vi "To Variant.vi"(0 "Obj in":refnum<class "Channel.lvclass">, 11 "error in (no error)":errorcluster) -> (4 "Obj out":refnum<class "Channel.lvclass">, 8 "Array":variant[](array[variant]), 15 "error out":errorcluster)   [LabVIEW 2020, in "Channel.lvclass"]
uses:
  Channel.lvclass
  Channel.lvclass/Channel.ctl
  Koop/KObject Class/KObject.lvclass
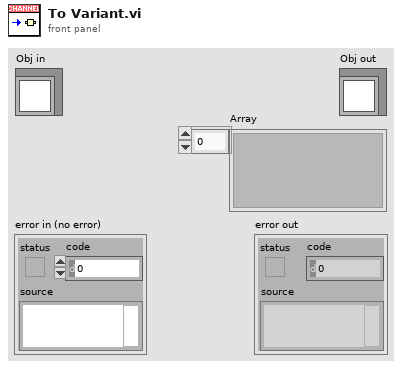
[diagram p1: front panel]
types:
  T1 = typedef "Channel.lvclass/Serialized.ctl" = cluster{"Name":string, "Destination":string, "AltPol":bool, "Persist":bool, "Waveform":refnum<class "Waveform.lvclass">, "Gate":refnum<class "Gate.lvclass">, "Level":refnum<class "Level.lvclass">, "AM":refnum<class "AM.lvclass">, "Filter":refnum<class "Filter.lvclass">, "Invert":bool, "Fade in":dbl, "Fade out":dbl}
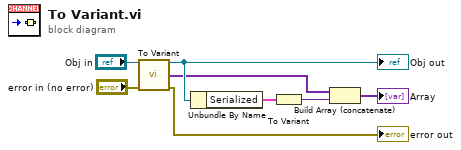
[diagram p0: block diagram]
diagram:
  n1 = call-parent "To Variant.vi"("KObject in"="Obj in", "error in (no error)"="error in (no error)") -> ("KObject out"=w3:refnum<class "Channel.lvclass">, "Array"=w2:variant[], "error out"=→"error out":errorcluster)  [unwired: 11 in]
  "Obj out" <- w3
  n2 = Unbundle By Name(w3) -> ("Serialized"=w4:T1)
  n3 = To Variant(anything=w4) -> (Variant=w5:variant)
  n4 = Build Array (concatenate)(w2, w5) -> (→"Array":variant[])
